vi "Read Data from  Waveform.vi"() -> ()   [LabVIEW 2011]
uses:
  Program Files (x86)/National Instruments/LabVIEW 2017/instr.lib/Agilent E5052X/Agilent E5052X.lvlib
panel:
  in  "error in (no error)":errorcluster
  out "error out":errorcluster
  out "X-Values":dbl[](array[numeric]) format="%^#_9g"
  out "Measurements":dbl[](array[numeric]) format="%^#_9g"
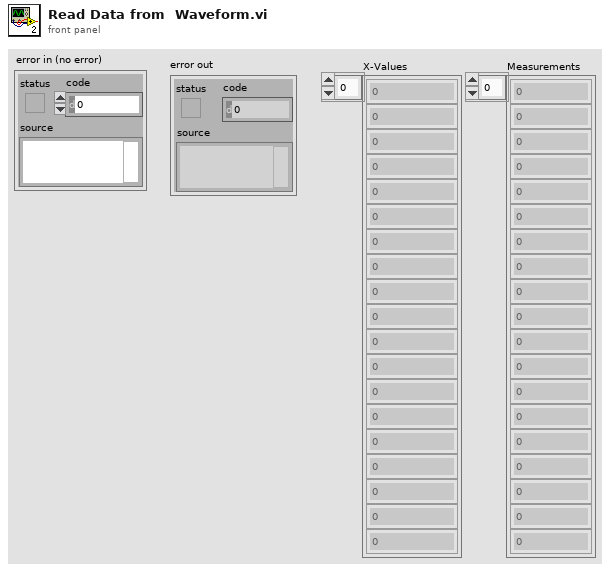
[diagram p1: front panel]
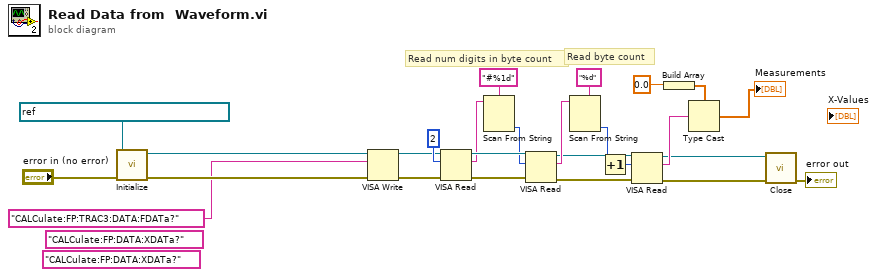
[diagram p0: block diagram]
diagram:
  (unwired) "CALCulate:FP:DATA:XDATa?" ("write buffer")
  (unwired) "CALCulate:FP:DATA:XDATa?" ("write buffer")
  # "Read num digits in byte count"
  # "Read byte count"
  n1 = call "Initialize.vi"("error in (no error)"="error in (no error)", "VISA resource name"=refnum<visa-resource-name> "TCPIP0::192.168.1.100::inst0::INSTR") -> ("error out"=w22:errorcluster, "VISA resource name out"=w23:refnum<visa-resource-name>)  [unwired: 8 in]
  n2 = VISA Write(VISA resource name=w23, write buffer="CALCulate:FP:TRAC3:DATA:FDATa?", error in (no error)=w22) -> (VISA resource name out=w5:refnum<visa-resource-name>, error out=w4:errorcluster)  [unwired: 1 out]
  n3 = VISA Read(VISA resource name=w5, byte count=u32 2, error in (no error)=w4) -> (VISA resource name out=w18:refnum<visa-resource-name>, read buffer=w14:string, error out=w19:errorcluster)  [unwired: 1 out]
  n4 = Scan From String(format string="#%1d", input string=w14) -> (output 1=w17:i32)  [unwired: 3 in, 3 out]
  n5 = VISA Read(VISA resource name=w18, byte count=w17, error in (no error)=w19) -> (VISA resource name out=w12:refnum<visa-resource-name>, read buffer=w16:string, error out=w11:errorcluster)  [unwired: 1 out]
  n6 = Scan From String(format string="%d", input string=w16) -> (output 1=w13:i32)  [unwired: 3 in, 3 out]
  n7 = Increment(x=w13) -> (x+1=w3:i32)
  n8 = VISA Read(VISA resource name=w12, byte count=w3, error in (no error)=w11) -> (VISA resource name out=w7:refnum<visa-resource-name>, read buffer=w8:string, error out=w6:errorcluster)  [unwired: 1 out]
  n9 = Build Array(sgl 0.0) -> (w9:sgl[])
  n10 = Type Cast(type=w9, x=w8) -> (*(type *) &x=→"Measurements":sgl[])
  n11 = call "Close.vi"("error in (no error)"=w6, "VISA resource name"=w7) -> ("error out"=→"error out":errorcluster)  [unwired: 9 in]
